vi "Log Message.vi"(5 "Level":T1, 8 "error in (no error)":errorcluster, 9 "Actor Type.Name":string, 10 "Message":string, 11 "Application Log in":refnum<class "Application Log.lvclass">) -> (0 "error out":errorcluster, 3 "Application Log out":refnum<class "Application Log.lvclass">)   [LabVIEW 2016, in "Stream Log.lvlib" / "Application Log.lvclass"]
doc: "--\nCopyright © 2017 Composed SystemsI All rights reserved.\n\nAuthor: Jon McBee <jon.mcbee@composed.io>\n\nThis library is provided \"AS IS\" ,WITHOUT WARRANTIES OR\nCONDITIONS OF ANY KIND, either express or implied.\n\nComposed Systems -- composed.io\n\nStream 0.0.1.1\nJon McBee - Composed Systems\nCopyright (c) 2017, Composed Systems"
uses:
  <userlib>/Composed Systems/Stream/Log/Application Log/Application Log.lvclass
  <userlib>/Composed Systems/Stream/Log/Application Log/Log Level.ctl
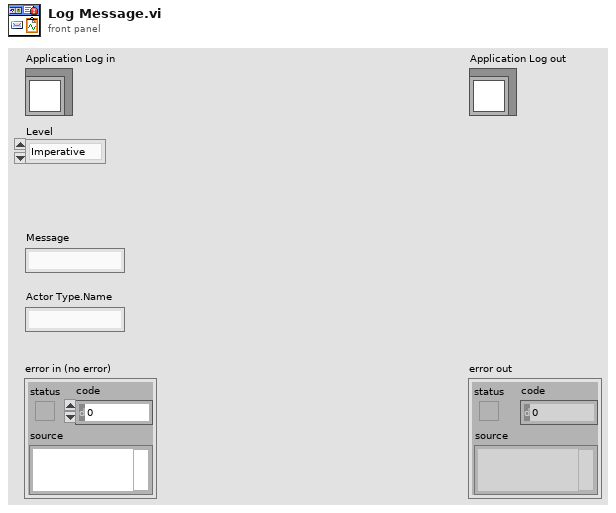
[diagram p1: front panel]
types:
  T1 = typedef "Stream Log.lvlib/Application Log.lvclass/Log Level.ctl" = enum16{"Imperative", "Major", "Minor", "Debug", "Off"}
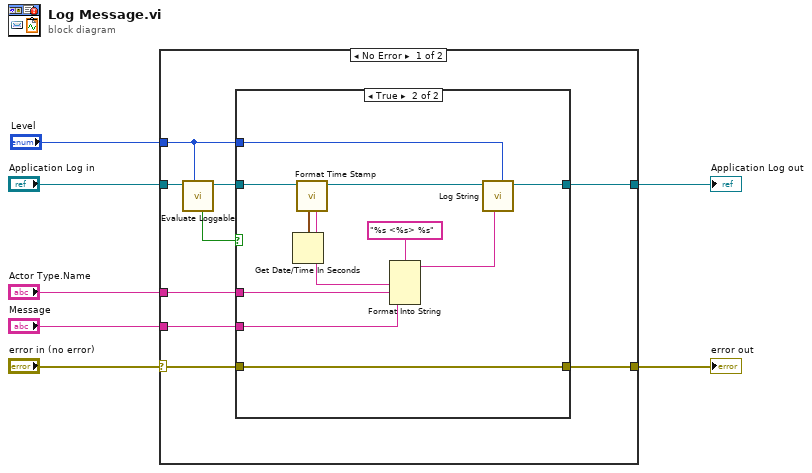
[diagram p0: block diagram]
diagram:
  n1 = case shown="No Error" "error in (no error)" {
    selector: "error in (no error)" -> [w14 w31]
    tunnel: [w10 w31] -> w6
    tunnel: [w12 w30] -> w4
    tunnel: "Application Log in" -> [w16 w30]
    tunnel: "Level" -> [w9 _]
    tunnel: "Message" -> [w15 _]
    tunnel: "Actor Type.Name" -> [w8 _]
    frame No Error {
      n2 = call <userlib>:"Evaluate Loggable.vi"("Level"=w9, "Application Log in"=w16) -> ("Application Log out"=w13:refnum<class "Application Log.lvclass">, "Log?"=w11:bool)  [unwired: 8 in]
      n3 = case shown="True" w11 {
        tunnel: w15 -> [_ w19]
        tunnel: w14 -> [w18 w26]
        tunnel: w13 -> [w17 w27]
        tunnel: [w17 w29] -> w12
        tunnel: [w18 w26] -> w10
        tunnel: w9 -> [_ w28]
        tunnel: w8 -> [_ w20]
        frame False {
        }
        frame True {
          n4 = Get Date/Time In Seconds() -> (seconds since 1Jan1904=w23:timestamp)
          n5 = call <userlib>:"Format Time Stamp.vi"("Time Stamp"=w23, "Application Log in"=w27) -> ("Application Log out"=w25:refnum<class "Application Log.lvclass">, "Formatted Time Stamp"=w22:string)  [unwired: 7 in, 1 out]
          n6 = Format Into String(format string="%s <%s> %s", w22, w20, w19) -> (resulting string=w21:string)  [unwired: 2 in, 1 out]
          n7 = call-dynamic "Log String.vi"("Level"=w28, "String"=w21, "Application Log in"=w25) -> ("Application Log out"=w29:refnum<class "Application Log.lvclass">)  [unwired: 7 in, 1 out]
        }
      }
    }
    frame Error {
    }
  }
  "error out" <- w6
  "Application Log out" <- w4
